vi "Disable RF Power.vi"(8 "error in (no error)":errorcluster, 11 "Comdel in":refnum<class "PL Comdel CX.lvclass">) -> (0 "error out":errorcluster, 3 "Comdel out":refnum<class "PL Comdel CX.lvclass">)   [LabVIEW 2015, in "PL Comdel CX.lvclass"]
doc: "Disables RF power."
uses:
  PL Comdel CX.lvclass
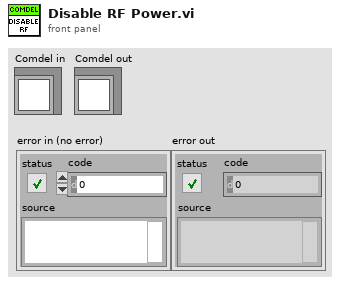
[diagram p1: front panel]
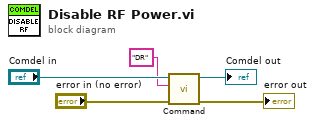
[diagram p0: block diagram]
diagram:
  n1 = call "Command.vi"("error in (no error)"="error in (no error)", "command"="DR", "Comdel in"="Comdel in") -> ("error out"=→"error out":errorcluster, "Comdel out"=→"Comdel out":refnum<class "PL Comdel CX.lvclass">)  [unwired: 6 in, 1 out]
